vi "stims2channels.vi"(10 "Stimulus channel array":bool[](array[boolean]), 11 "Stimuli":string) -> (3 "Stimulus channels":bool[](array[boolean]))   [LabVIEW 2014]
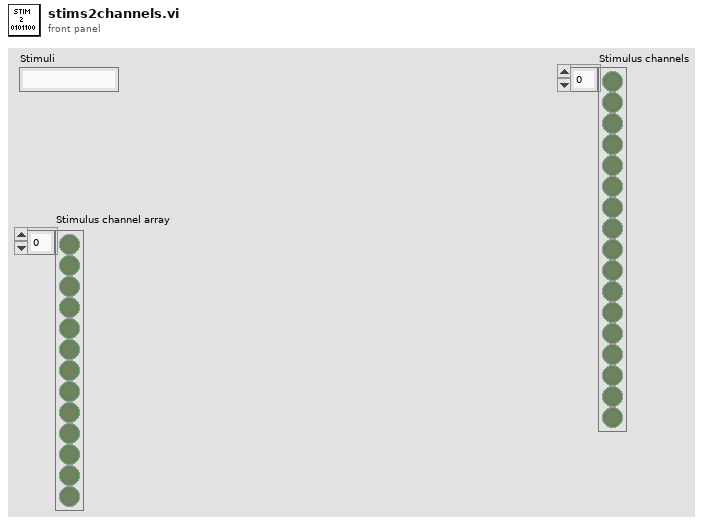
[diagram p1: front panel]
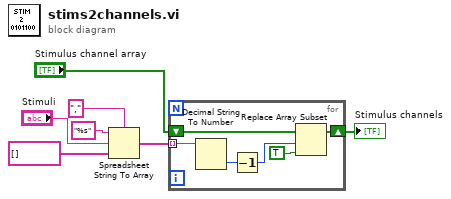
[diagram p0: block diagram]
diagram:
  n1 = Spreadsheet String To Array(delimiter (Tab)=",", format string="%s", spreadsheet string="Stimuli", array type (2D Dbl)=string[] []) -> (array=w3:string[])
  n2 = for {
    tunnel: w3 -> [w12] mode=indexing
    shift-right: [w8] -> w1
    shift-left: "Stimulus channel array" -> [w10]
    n3 = Decimal String To Number(string=w12) -> (number=w11:i32)  [unwired: 2 in, 1 out]
    n4 = Decrement(x=w11) -> (x-1=w13:i32)
    n5 = Replace Array Subset(array=w10, new element=TRUE ("new element/subarray"), index=w13) -> (w8:bool[])
  }
  "Stimulus channels" <- w1
